vi "set_state.vi"(8 "error in (no error)":errorcluster, 10 "state":bool, 11 "DAQmxDigitalOut in":refnum<class "DigitalOutDL110325DAQmx.lvclass">) -> (0 "error out":errorcluster, 3 "DAQmxDigitalOut out":refnum<class "DigitalOutDL110325DAQmx.lvclass">)   [LabVIEW 2010, in "DigitalOutDL110325DAQmx.lvclass"]
uses:
  DigitalOutDL110325DAQmx.lvclass
  DigitalOutDL110325DAQmx.lvclass/DigitalOutDL110325DAQmx.ctl
  <vilib>/DAQmx/write.llb/DAQmx Write (Digital Bool 1Line 1Point).vi
  <vilib>/daqmx/miscellaneous.llb/DAQmx Fill In Error Info.vi
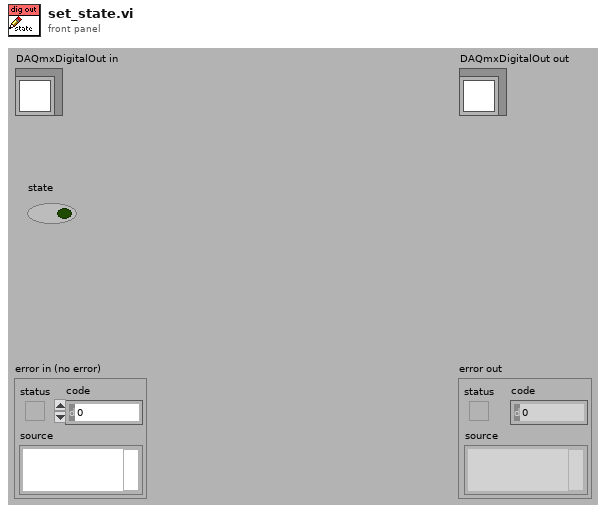
[diagram p1: front panel]
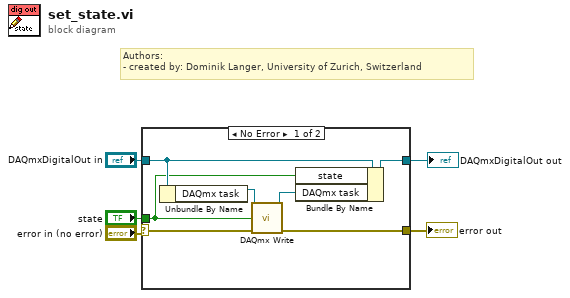
[diagram p0: block diagram]
diagram:
  # "Authors: \n- created by: Dominik Langer, University of Zurich, Switzerland"
  n1 = case shown="No Error" "error in (no error)" {
    selector: "error in (no error)" -> [w10 w14]
    tunnel: [w9 w14] -> w4
    tunnel: [w7 w13] -> w2
    tunnel: "DAQmxDigitalOut in" -> [w8 w13]
    tunnel: "state" -> [w6 _]
    frame No Error {
      n2 = Unbundle By Name(w8) -> ("DAQmx task"=w12:refnum<k21>)
      n3 = call-poly <vilib>:"DAQmx Write.vi"("task/channels in"=w12, "data"=w6, "error in"=w10) -> ("task out"=w11:refnum<k21>, "error out"=w9:errorcluster)  [unwired: 2 in, 9 out]
      n4 = Bundle By Name(cluster=w8, "state"=w6, "DAQmx task"=w11) -> (w7:refnum<class "DigitalOutDL110325DAQmx.lvclass">)
    }
    frame Error {
    }
  }
  "error out" <- w4
  "DAQmxDigitalOut out" <- w2
